vi "Cluster_to_Picture.vi"(6 "translation":cluster{"X":i32, "Y":i32}, 8 "viewer":enum16{"俯视图", "轴测图"}(ring), 9 "PicAjust":T3={"TranslationVector"=[], "scale"=1.0, "Pitch（x) "=0.0, "Yaw（y)"=0.0, "Roll（z) "=0.0} {"Roll（z)" scale=-90.0..90.0; "Yaw（y)" scale=-90.0..90.0; "Pitch（x)" scale=-90.0..90.0}, 10 "Cluster of 7 Type Data":T2(array[cluster]), 11 "Scalar":dbl=0.06) -> (3 "Anto Drawer":picture)   [LabVIEW 2014]
doc: "根据簇中数据画二维平面图"
uses:
  <vilib>/Analysis/Matrix/Datatypes/RealMatrix.ctl
  <vilib>/Analysis/Matrix/NI_Matrix.lvlib
panel:
  in  "Data Matrix":T1=[[0.0, 0.0, 0.0], [0.0, 11696.0, 0.0], [11414.5, 11843.9, 150.0], [14173.5, 5920.8, 150.0], [13501.3, 5521.4, 150.0]]
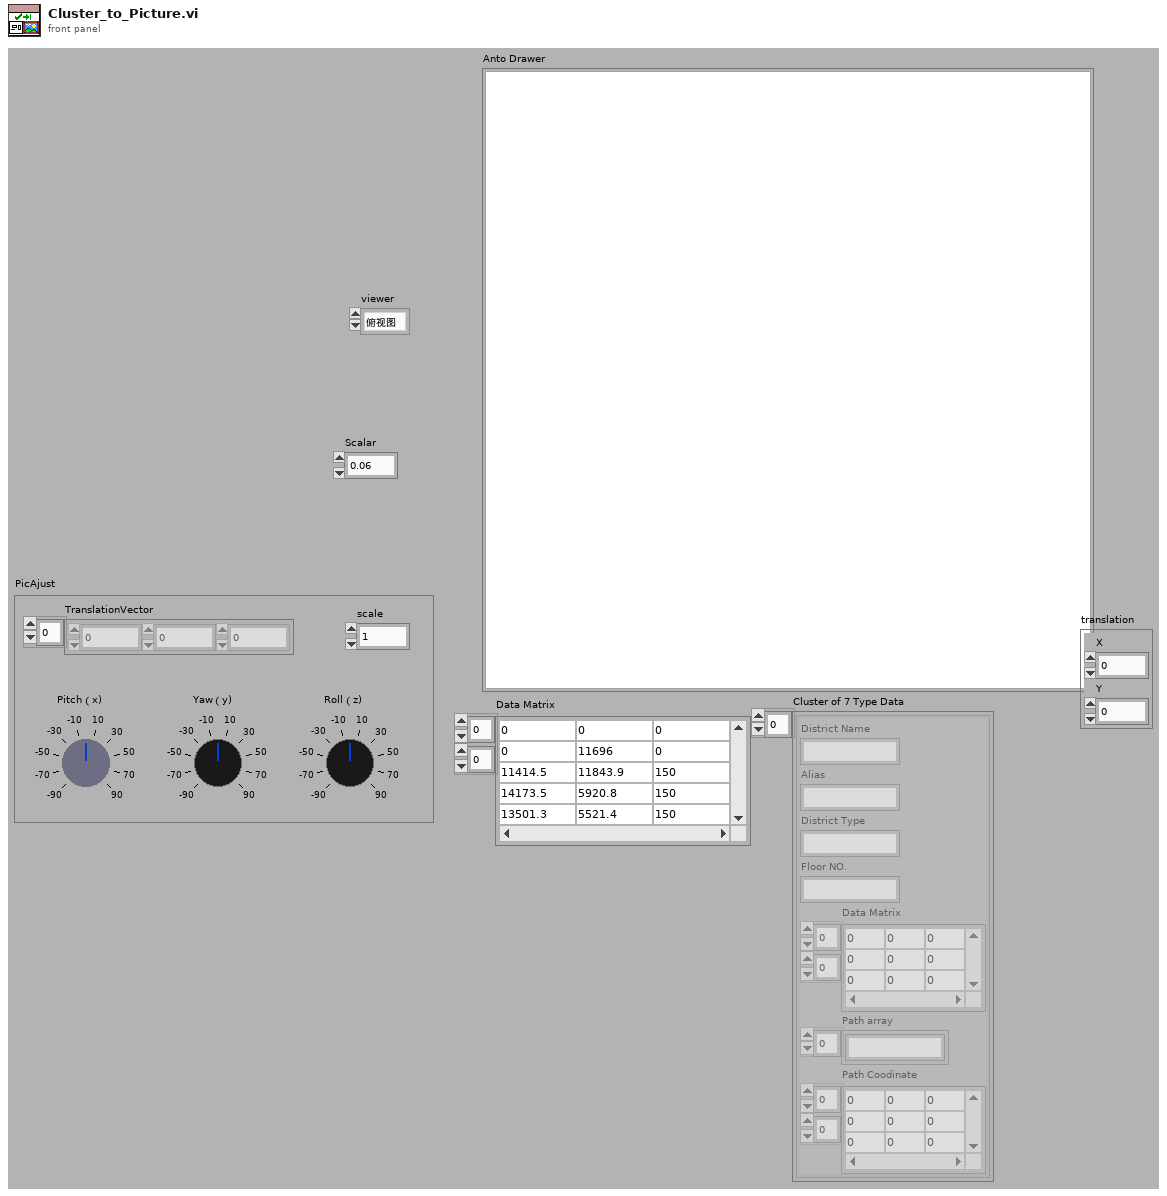
[diagram p1: front panel]
types:
  T1 = typedef "NI_Matrix.lvlib/RealMatrix.ctl" = dbl[][]
  T2 = cluster{"District Name":string, "Alias":string, "District Type":string, "Floor NO.":string, "Data Matrix":T1, "Path array":string[], "Path Coodinate":T1}[]
  T3 = cluster{"TranslationVector":dbl[], "scale":dbl, "Pitch（x) ":dbl, "Yaw（y)":dbl, "Roll（z) ":dbl}
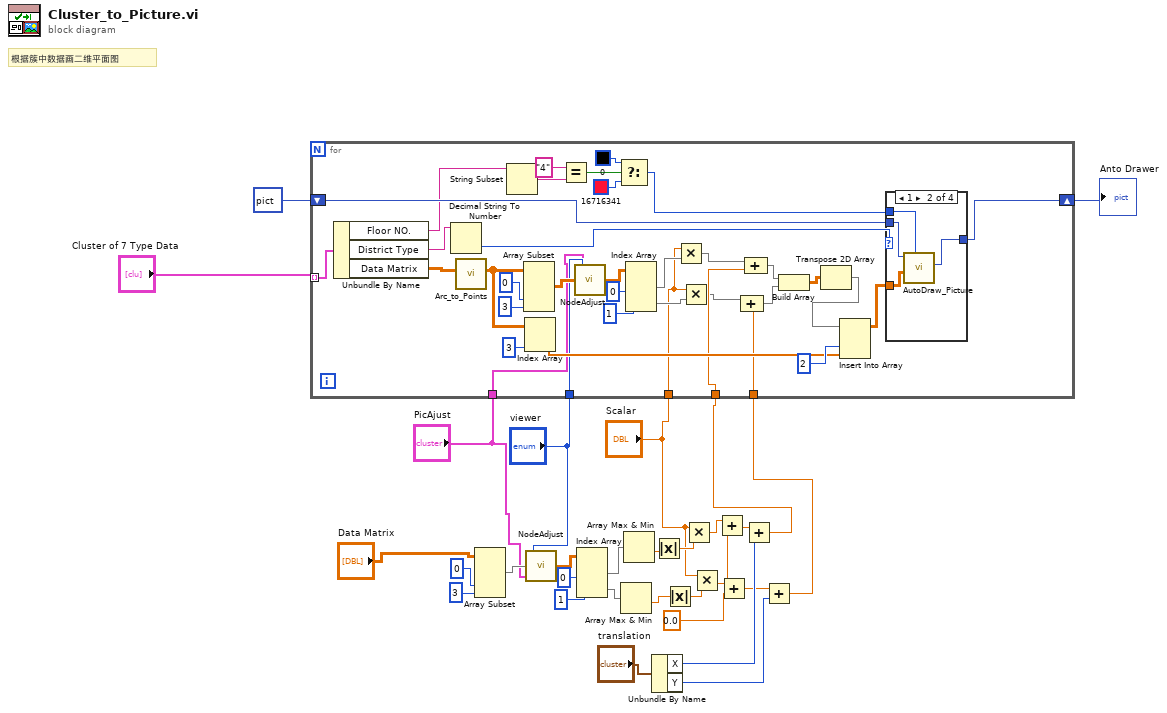
[diagram p0: block diagram]
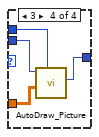
[diagram p4: hidden frame]
diagram:
  w10 = 0.0 ("y")
  # "根据簇中数据画二维平面图"
  n1 = Array Subset(array="Data Matrix", index (col)=0 ("索引"), length (col)=3 ("长度")) -> (w20:T1)  [unwired: 2 in]
  n2 = call "NodeAdjust.vi"("PicAjust"="PicAjust", "NodeM"=w20, "视图"="viewer") -> ("NewNodeM"=w23:dbl[][])
  n3 = Index Array(array=w23, index (col) #1=0 ("禁用的索引 (列)"), index (col) #2=1 ("索引 (列)")) -> (element #1=w27:dbl[], element #2=w26:dbl[])  [unwired: 2 in]
  n4 = Array Max & Min(array=w26) -> (min value=w13:dbl)  [unwired: 3 out]
  n5 = Array Max & Min(array=w27) -> (min value=w18:dbl)  [unwired: 3 out]
  n6 = Unbundle By Name("translation") -> ("X"=w5:i32, "Y"=w2:i32)
  n7 = Absolute Value(x=w18) -> (abs(x)=w17:dbl)
  n8 = Absolute Value(x=w13) -> (abs(x)=w14:dbl)
  n9 = Multiply(x="Scalar", y=w17) -> (x*y=w16:dbl)
  n10 = Multiply(x="Scalar", y=w14) -> (x*y=w11:dbl)
  n11 = Add(x=w16, y=w10) -> (x+y=w6:dbl)
  n12 = Add(x=w11, y=w10) -> (x+y=w3:dbl)
  n13 = Add(x=w6, y=w5) -> (x+y=w4:dbl)
  n14 = Add(x=w3, y=w2) -> (x+y=w1:dbl)
  n15 = for {
    tunnel: "Cluster of 7 Type Data" -> [w66] mode=indexing
    shift-right: [w53] -> w28
    shift-left: picture data[5B] ("Init Picture") -> [w54]
    tunnel: "viewer" -> [w48]
    tunnel: w4 -> [w47]
    tunnel: w1 -> [w46]
    tunnel: "Scalar" -> [w38]
    tunnel: "PicAjust" -> [w37]
    n16 = Unbundle By Name(w66) -> ("Floor NO."=w36:string, "District Type"=w63:string, "Data Matrix"=w65:T1)
    n17 = Decimal String To Number(string=w63) -> (number=w62:i32)  [unwired: 2 in, 1 out]
    n18 = call "Arc_to_Points.vi"("Data Matrix"=w65) -> ("Points of Data Matrix"=w61:dbl[][])  [unwired: 10 in]
    n19 = String Subset ("截取字符串")(string=w36) -> (substring=w35:string)  [unwired: 2 in]
    n20 = Array Subset(array=w61, index (col)=0 ("索引"), length (col)=3 ("长度")) -> (w64:dbl[][])  [unwired: 2 in]
    n21 = Index Array(array=w61, index (col)=3 ("禁用的索引 (列)")) -> (element=w56:dbl[])  [unwired: 1 in]
    n22 = Equal?(x="4", y=w35) -> (x = y?=w33:bool)
    n23 = call "NodeAdjust.vi"("PicAjust"=w37, "NodeM"=w64, "视图"=w48) -> ("NewNodeM"=w52:dbl[][])
    n24 = Select(t=u32 0 ("color(black)"), s=w33, f=u32 16716341 ("color(black)")) -> (s? t:f=w32:u32)
    n25 = Index Array(array=w52, index (col) #1=0 ("禁用的索引 (列)"), index (col) #2=1 ("索引 (列)")) -> (element #1=w45:dbl[], element #2=w43:dbl[])  [unwired: 2 in]
    n26 = Multiply(x=w38, y=w45) -> (x*y=w44:dbl[])
    n27 = Multiply(x=w38, y=w43) -> (x*y=w42:dbl[])
    n28 = Compound Arithmetic op=ADD(w42, w46) -> (w40:dbl[])
    n29 = Compound Arithmetic op=ADD(w44, w47) -> (w41:dbl[])
    n30 = Build Array(w41, w40) -> (w39:dbl[][])
    n31 = Transpose 2D Array(2D array=w39) -> (transposed array=w49:dbl[][])
    n32 = Insert Into Array(array=w49, index (col)=2 ("禁用的索引 (列)"), new element=w56) -> (w55:dbl[][])  [unwired: 1 in]
    n33 = case shown="1" w62 {
      tunnel: w55 -> [_ w71 _ w76]
      tunnel: [w67 w70 w72 w74] -> w53
      tunnel: w54 -> [w67 w69 w72 w75]
      tunnel: w32 -> [_ w68 _ w73]
      frame 0, Default {
      }
      frame 1 {
        n34 = call "AutoDraw_Picture.vi"("color(black)"=w68, "Data Array for Picture"=w71, "Init Picture"=w69) -> ("Anto Drawer"=w70:picture)  [unwired: 8 in]
      }
      frame 2 {
      }
      frame 3 {
        n35 = call "AutoDraw_Picture.vi"("color(black)"=w73, "Data Array for Picture"=w76, "Init Picture"=w75) -> ("Anto Drawer"=w74:picture)  [unwired: 8 in]
      }
    }
  }
  "Anto Drawer" <- w28
